vi "string.vi"(1 "String 2 in":string, 2 "String 1 in":string) -> (0 "Concatenated Strings out":string)   [LabVIEW 2010]
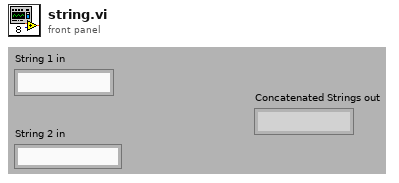
[diagram p1: front panel]
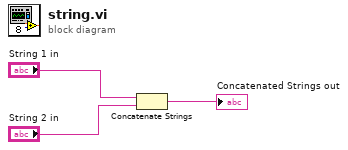
[diagram p0: block diagram]
diagram:
  n1 = Concatenate Strings("String 1 in", "String 2 in") -> (→"Concatenated Strings out":string)
